vi "Open Explorer Window.vi"() -> ()   [LabVIEW 2013]
panel:
  out "resulting string":string
  out "error out":errorcluster
  in  "Path":path
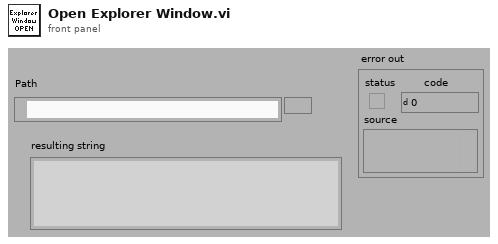
[diagram p1: front panel]
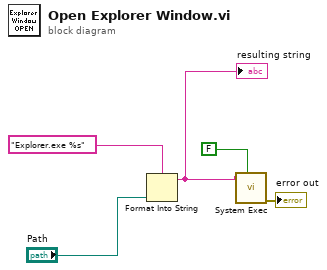
[diagram p0: block diagram]
diagram:
  n1 = Format Into String(format string="Explorer.exe %s" ("command line"), "Path") -> (resulting string=w2:string)  [unwired: 2 in, 1 out]
  "resulting string" <- w2
  n2 = call <vilib>:"System Exec.vi"("wait until completion? (T)"=FALSE, "command line"=w2) -> ("error out"=→"error out":errorcluster)  [unwired: 6 in, 3 out]
